vi "Create Message Setter (from Template).vi"(8 "error in (no error)":errorcluster, 10 "RPC Message Name":string, 11 "RPC Messages Folder (ProjectItem) in":refnum<vi>) -> (0 "error out":errorcluster, 1 "Created?":bool, 2 "VI out":refnum<vi>, 3 "RPC Messages Folder (ProjectItem) out":refnum<vi>)   [LabVIEW 2019, in "gRPC Scripting Tools.lvlib"]
uses:
  gRPC Scripting Tools.lvlib
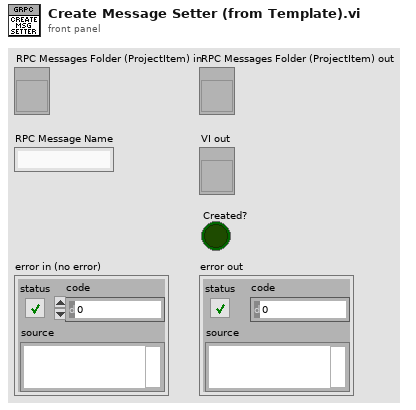
[diagram p1: front panel]
types:
  T1 = enum32{"invalid VI type", "Standard VI", "Control VI", "Global VI", "Polymorphic VI", "Configuration VI", "SubSystem", "Facade VI", "Method VI"}
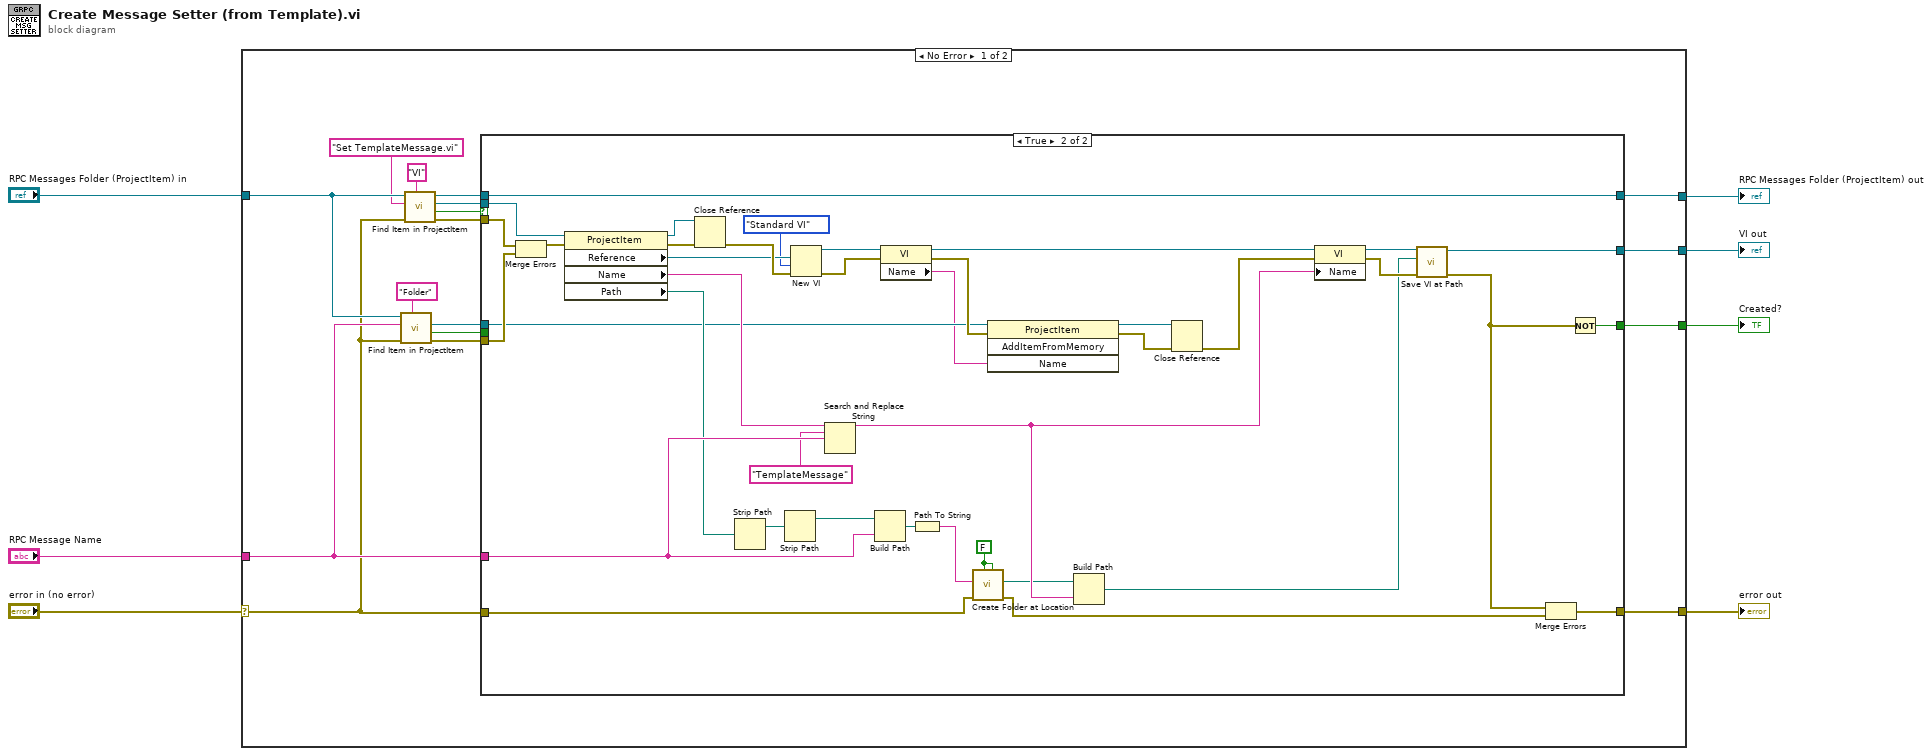
[diagram p0: block diagram]
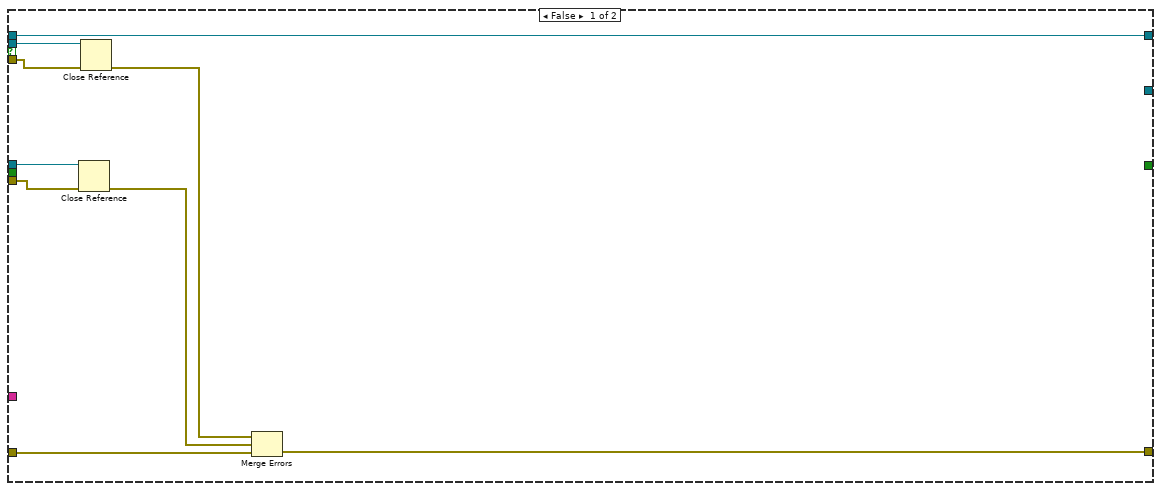
[diagram p2: hidden frame]
diagram:
  n1 = case shown="No Error" "error in (no error)" {
    selector: "error in (no error)" -> [w13 w73]
    tunnel: "RPC Message Name" -> [w24 _]
    tunnel: "RPC Messages Folder (ProjectItem) in" -> [w23 w74]
    tunnel: [w22 w73] -> w5
    tunnel: [w10 w74] -> w4
    tunnel: [w19 _] -> w3
    tunnel: [w9 _] -> w1
    frame No Error {
      n2 = call "Find Item in ProjectItem.vi"("Item Type"="Folder", "error in (no error)"=w13, "Name"=w24, "ProjectItem in"=w23) -> ("error out"=w21:errorcluster, "Found ?"=w8:bool, "Item Refnum out"=w18:refnum<vi>)  [unwired: 4 in, 1 out]
      n3 = call "Find Item in ProjectItem.vi"("Item Type"="VI", "error in (no error)"=w13, "Name"="Set TemplateMessage.vi", "ProjectItem in"=w23) -> ("error out"=w20:errorcluster, "Found ?"=w12:bool, "Item Refnum out"=w17:refnum<vi>, "ProjectItem out"=w11:refnum<vi>)  [unwired: 4 in]
      n4 = case shown="True" w12 {
        tunnel: w24 -> [_ w72]
        tunnel: [w25 w68] -> w22
        tunnel: w21 -> [w32 w66]
        tunnel: w20 -> [w29 w64]
        tunnel: [_ w62] -> w19
        tunnel: w18 -> [w31 w47]
        tunnel: w17 -> [w30 w41]
        tunnel: w13 -> [w26 w40]
        tunnel: w11 -> [w33 w39]
        tunnel: [w33 w39] -> w10
        tunnel: [_ w34] -> w9
        tunnel: w8 -> [_ _]
        frame False {
          n5 = Close Reference(reference=w31, error in (no error)=w32) -> (error out=w28:errorcluster)
          n6 = Close Reference(reference=w30, error in (no error)=w29) -> (error out=w27:errorcluster)
          n7 = Merge Errors(w27, w28, w26) -> (w25:errorcluster)
        }
        frame True {
          w63 = FALSE ("Use Relative (F)")
          n8 = Merge Errors(w64, w66) -> (w65:errorcluster)
          n9 = property class="ProjectItem"(reference=w41, error in=w65) -> (reference out=w71:refnum<vi>, error out=w69:errorcluster, "Reference"=w45:refnum<vi>, "Name"=w54:string, "Path"=w52:path)
          n10 = Close Reference(reference=w71, error in (no error)=w69) -> (error out=w70:errorcluster)
          n11 = Strip Path(path=w52) -> (stripped path=w48:path)  [unwired: 1 out]
          n12 = Strip Path(path=w48) -> (stripped path=w49:path)  [unwired: 1 out]
          n13 = New VI(8:w70, 9:T1."Standard VI" ("vi type (standard vi)"), 10:w45) -> (0:w44:errorcluster, 3:w42:refnum<vi>)  [unwired: 1 in, 3 out]
          n14 = Search and Replace String(input string=w54, search string="TemplateMessage", replace string=w72) -> (result string=w58:string)  [unwired: 5 in, 3 out]
          n15 = Build Path(base path=w49, name or relative path=w72) -> (appended path=w50:path)
          n16 = property class="VI"(reference=w42, error in=w44) -> (reference out=w55:refnum<vi>, error out=w56:errorcluster, "Name"=w46:string)
          n17 = Path To String(path=w50) -> (string=w51:string)
          n18 = call "Create Folder at Location.vi"("Override existing (F)"=w63, "Use Relative (F)"=w63, "Error In"=w40, "Path"=w51) -> ("Error Out"=w67:errorcluster, "Full path out"=w57:path)  [unwired: 5 in, 1 out]
          n19 = invoke class="ProjectItem" method="AddItemFromMemory"(reference=w47, error in=w56, "Name"=w46) -> (reference out=w37:refnum<vi>, error out=w38:errorcluster)  [unwired: 1 in, 2 out]
          n20 = Build Path(base path=w57, name or relative path=w58) -> (appended path=w60:path)
          n21 = Close Reference(reference=w37, error in (no error)=w38) -> (error out=w36:errorcluster)
          n22 = property class="VI"(reference=w55, error in=w36, "Name"=w58) -> (reference out=w59:refnum<vi>, error out=w61:errorcluster)
          n23 = call "Save VI at Path.vi"("error in (no error)"=w61, "Path"=w60, "VI in"=w59) -> ("error out"=w35:errorcluster, "VI out"=w62:refnum<vi>)  [unwired: 6 in, 1 out]
          n24 = Merge Errors(w35, w67) -> (w68:errorcluster)
          n25 = Not(x=w35) -> (.not. x?=w34:bool)
        }
      }
    }
    frame Error {
    }
  }
  "error out" <- w5
  "RPC Messages Folder (ProjectItem) out" <- w4
  "VI out" <- w3
  "Created?" <- w1
